vi "Initialize.vi"(8 "error in (no error)":errorcluster, 11 "socket REP in":refnum<class "socket REP.lvclass">) -> (0 "error out":errorcluster, 3 "socket REP out":refnum<class "socket REP.lvclass">)   [LabVIEW 2018, in "socket REP.lvclass"]
uses:
  socket REP.lvclass
  C:/Users/orlando/Documents/Orlando/communication-manager/communication-manager/Socket/Socket.lvclass
  Socket/Socket.lvclass
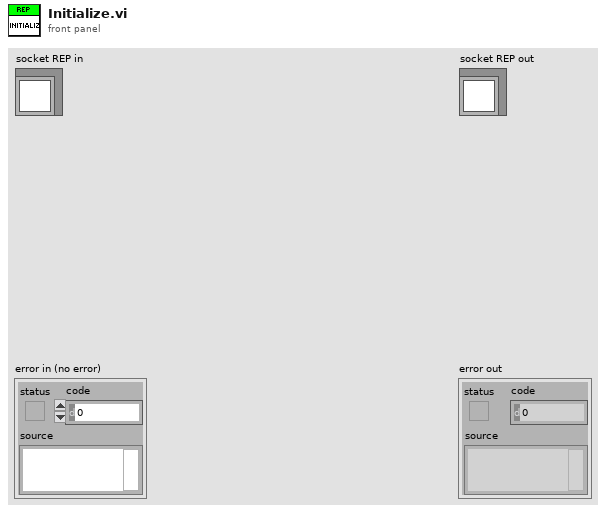
[diagram p1: front panel]
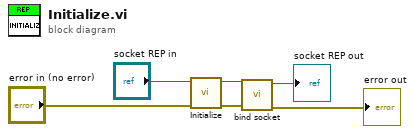
[diagram p0: block diagram]
diagram:
  n1 = call-parent "Initialize.vi"("error in (no error)"="error in (no error)", "Socket in"="socket REP in") -> ("error out"=w3:errorcluster, "Socket out"=w4:refnum<class "socket REP.lvclass">)  [unwired: 8 in]
  n2 = call "bind socket.vi"("error in (no error)"=w3, "Socket in"=w4) -> ("error out"=→"error out":errorcluster, "Socket out"=→"socket REP out":refnum<class "socket REP.lvclass">)  [unwired: 8 in]
